vi "Grab.vi"(8 "error in (no error)":errorcluster, 10 "Image":T1, 11 "Recipe Test Sim Camera Driver in":refnum<class "Recipe Test Sim Camera Driver.lvclass">) -> (0 "error out":errorcluster, 2 "Image out":T1, 3 "Recipe Test Sim Camera Driver out":refnum<class "Recipe Test Sim Camera Driver.lvclass">)   [LabVIEW 2022 SP3, in "Recipe Test Sim Camera Driver.lvclass"]
uses:
  Recipe Test Sim Camera Driver.lvclass
  Recipe Test Sim Camera Driver.lvclass/Recipe Test Sim Camera Driver.ctl
  Sim Camera Driver/Sim Camera Driver.lvclass
  <vilib>/Utility/file.llb/Read Delimited Spreadsheet (I64).vi
  Laser/Test Station SIM Laser Driver/Test Station SIM Laser Driver.lvclass
  Laser/Test Station SIM Laser Driver/Action.ctl
  C:/XY Stage/Camera/Sim Camera Driver/Sim Camera Driver.lvclass
  C:/XY Stage/XY Stage/Framework/Base/Base.lvclass
  C:/XY Stage/Camera/Camera Driver/Camera Driver.lvclass
  C:/XY Stage/Camera/Test Recipe Sim Camera Driver/Recipe Test Sim Camera Driver.lvclass
  <vilib>/vision/Image Controls.llb/IMAQ Image.ctl
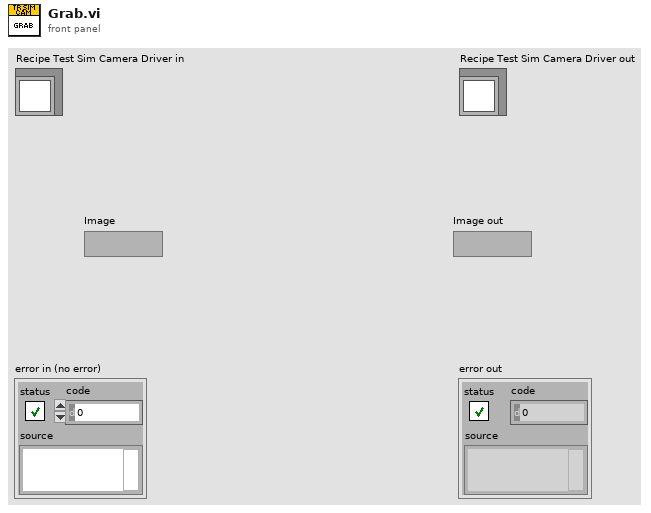
[diagram p1: front panel]
types:
  T1 = typedef "IMAQ Image.ctl" = refnum<image>
  T2 = typedef "Test Station SIM Laser Driver.lvclass/Action.ctl" = enum16{"Read Data", "Set Data"}
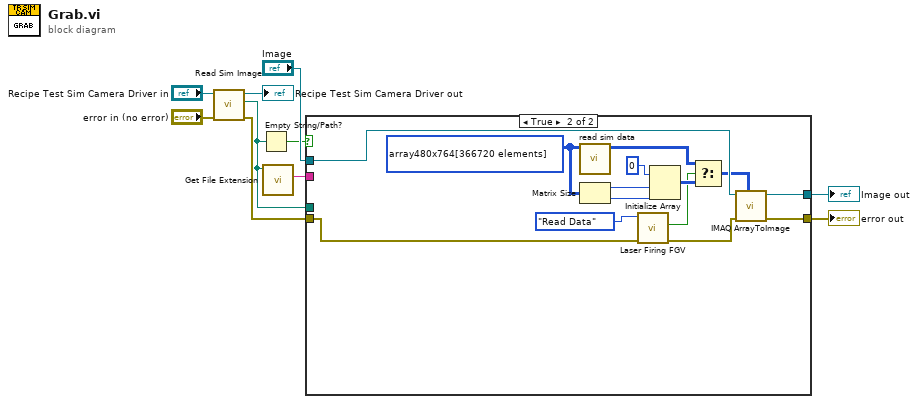
[diagram p0: block diagram]
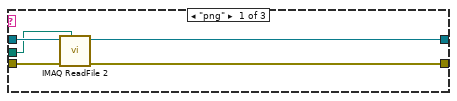
[diagram p3: hidden frame]
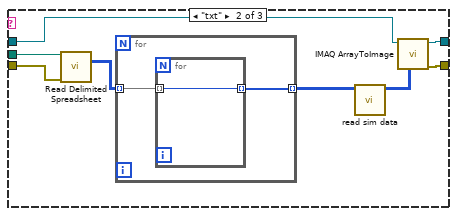
[diagram p4: hidden frame]
diagram:
  n1 = call "Read Sim Image.vi"("error in (no error)"="error in (no error)", "Sim Camera Driver in"="Recipe Test Sim Camera Driver in") -> ("error out"=w1:errorcluster, "Sim Image"=w4:path, "Sim Camera Driver out"=→"Recipe Test Sim Camera Driver out":refnum<class "Recipe Test Sim Camera Driver.lvclass">)  [unwired: 7 in]
  n2 = Empty String/Path?(string/path=w4) -> (empty?=w7:bool)
  n3 = call <vilib>:"Get File Extension.vi"("file"=w4) -> ("lowercase file extension"=w6:string)  [unwired: 6 in, 4 out]
  n4 = case shown="True" w7 {
    tunnel: "Image" -> [w16 w46]
    tunnel: [w15 w48] -> w9
    tunnel: w6 -> [w14 _]
    tunnel: [w13 w47] -> w10
    tunnel: w4 -> [w12 _]
    tunnel: w1 -> [w11 w35]
    frame False {
      n5 = case shown="Default" w14 {
        tunnel: w11 -> [w18 w29 w33]
        tunnel: w12 -> [w20 w28 _]
        tunnel: w16 -> [w21 w26 w34]
        tunnel: [w17 w25 w33] -> w13
        tunnel: [w19 w24 w34] -> w15
        frame "png" {
          n6 = call "IMAQ ReadFile 2"("File Path"=w20, "error in (no error)"=w18, "Image"=w21) -> ("error out"=w17:errorcluster, "Image Out"=w19:T1)  [unwired: 4 in, 3 out]
        }
        frame "txt" {
          n7 = call-poly <vilib>:"Read Delimited Spreadsheet.vi"("file path (dialog if empty)"=w28, "error in (no error)"=w29) -> ("all rows"=w23:i64[][])  [unwired: 8 in, 5 out]
          n8 = for {
            tunnel: w23 -> [w31] mode=indexing
            tunnel: [w30] -> w22 mode=indexing
            n9 = for {
              tunnel: w31 -> [w32] mode=indexing
              tunnel: [w32] -> w30 mode=indexing
            }
          }
          n10 = call "read sim data.vi"("Array IN"=w22) -> ("Array Out"=w27:u16[][])  [unwired: 10 in]
          n11 = call "IMAQ ArrayToImage"("Image Pixels (Float)"=w27, "Image"=w26) -> ("error out"=w25:errorcluster, "Image Out"=w24:T1)  [unwired: 8 in]
        }
        frame Default {
        }
      }
    }
    frame True {
      w45 = u16[][] array480x764[366720 elements] ("Array")
      n12 = call "read sim data.vi"("Array IN"=w45) -> ("Array Out"=w41:u16[][])  [unwired: 10 in]
      n13 = Matrix Size(0:w45) -> (1:w44:i32, 2:w43:i32)
      n14 = call "Laser Firing FGV.vi"("error in (no error)"=w35, "Action"=Action."Read Data") -> ("error out"=w36:errorcluster, "Laser Firing"=w38:bool)  [unwired: 8 in]
      n15 = Initialize Array(u16 0, w44, w43) -> (w40:u16[][])
      n16 = Select(t=w41, s=w38, f=w40) -> (s? t:f=w39:u16[][])
      n17 = call "IMAQ ArrayToImage"("Image Pixels (U16)"=w39, "error in (no error)"=w36, "Image"=w46) -> ("error out"=w47:errorcluster, "Image Out"=w48:T1)  [unwired: 7 in]
    }
  }
  "error out" <- w10
  "Image out" <- w9
